vi "Digital_Output_8Channels.vi"(1 "States":bool[](array[boolean])=[FALSE, FALSE, FALSE, FALSE, FALSE, FALSE, FALSE, FALSE], 2 "IO":T1={"DO 0"="Mod1/DIO2", "DO 1"="Mod1/DIO2", "DO 2"="Mod1/DIO2", "DO 3"="Mod1/DIO2", "DO 4"="Mod1/DIO2", "DO 5"="Mod1/DIO2", "DO 6"="Mod1/DIO2", "DO 7"="Mod1/DIO2"}) -> ()   [LabVIEW 2015]
uses:
  <vilib>/eio/EIONode/EIONode.xnode
  <vilib>/rvi/eio/common/nirviEmuTemplateMethod_errors.vi
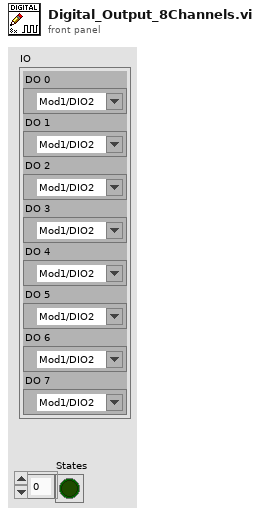
[diagram p1: front panel]
types:
  T1 = cluster{"DO 0":refnum<k21>, "DO 1":refnum<k21>, "DO 2":refnum<k21>, "DO 3":refnum<k21>, "DO 4":refnum<k21>, "DO 5":refnum<k21>, "DO 6":refnum<k21>, "DO 7":refnum<k21>}
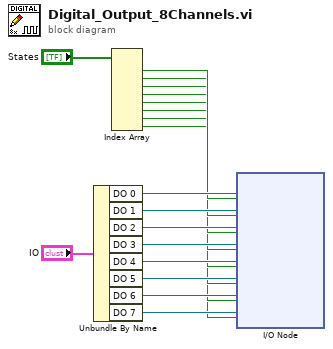
[diagram p0: block diagram]
diagram:
  n1 = Unbundle By Name("IO") -> ("DO 0"=w17:refnum<k21>, "DO 1"=w16:refnum<k21>, "DO 2"=w15:refnum<k21>, "DO 3"=w14:refnum<k21>, "DO 4"=w13:refnum<k21>, "DO 5"=w12:refnum<k21>, "DO 6"=w11:refnum<k21>, "DO 7"=w10:refnum<k21>)
  n2 = Index Array(array="States") -> (element #1=w8:bool, element #2=w7:bool, element #3=w6:bool, element #4=w5:bool, element #5=w4:bool, element #6=w3:bool, element #7=w2:bool, element #8=w1:bool)  [unwired: 8 in]
  n3 = xnode "I/O Node"("I/O Item"=w8, "FPGA I/O In"=w17, "I/O Item"=w7, "FPGA I/O In"=w16, "I/O Item"=w6, "FPGA I/O In"=w15, "I/O Item"=w5, "FPGA I/O In"=w14, "I/O Item"=w4, "FPGA I/O In"=w13, "I/O Item"=w3, "FPGA I/O In"=w12, "I/O Item"=w2, "FPGA I/O In"=w11, "I/O Item"=w1, "FPGA I/O In"=w10) -> ()  [unwired: 8 out]
